vi "test.vi"() -> ()   [LabVIEW 2017]
uses:
  <vilib>/Analysis/NI_AALBase.lvlib
panel:
  out "Цифровой сигнал с паузами 3":dbl[][](graph)
  in  "Кол-во выборок":i32=400
  in  "Циклов в секунду\n(Модуляция)":i32(slide) scale=0.0..10.0
  out "Цифровой сигнал с паузами 2":dbl[][](graph)
  out "Waveform Graph":dbl[](graph)
  in  "Количество бит":i32=8
  out "Биты на выходе 1":dbl[](array[numeric])
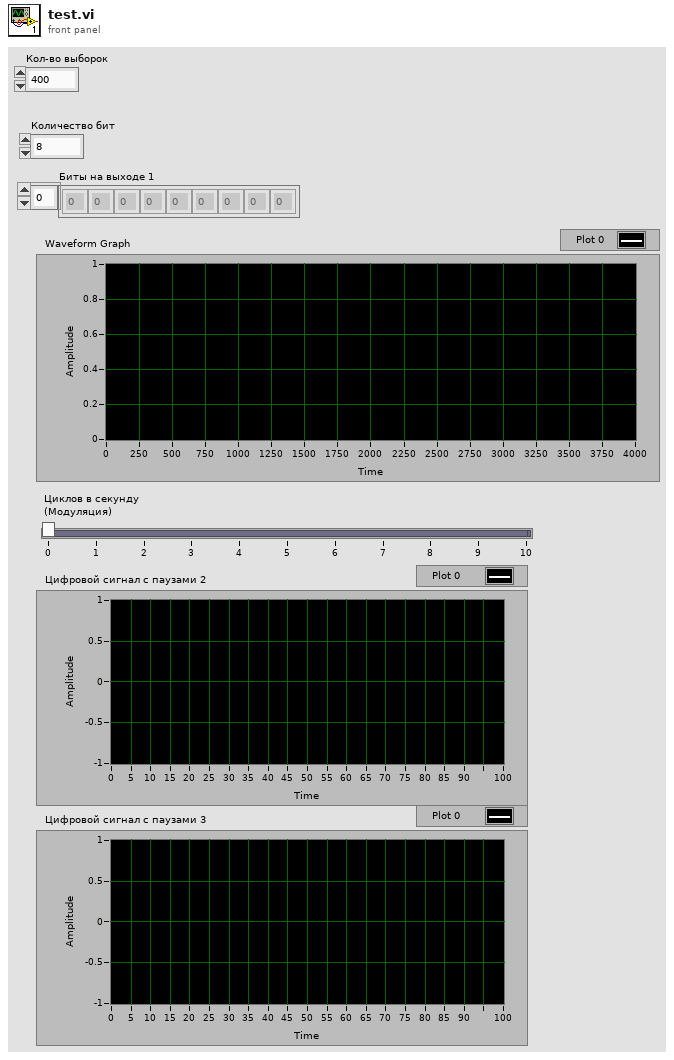
[diagram p1: front panel]
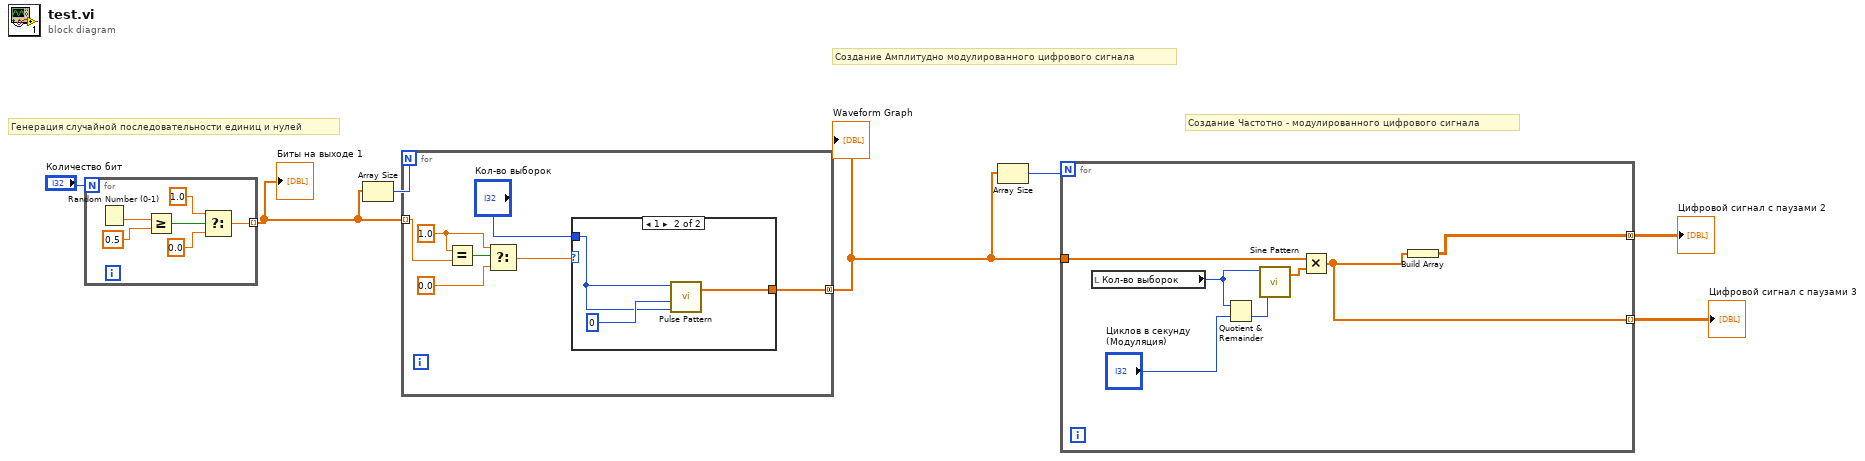
[diagram p0: block diagram]
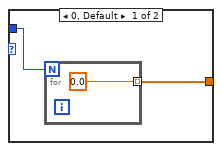
[diagram p2: hidden frame]
diagram:
  # "Создание Частотно - модулированного цифрового сигнала"
  # "Создание Амплитудно модулированного цифрового сигнала"
  # "Генерация случайной последовательности единиц и нулей"
  n1 = for {
    N: "Количество бит" -> [_]
    tunnel: [w8] -> w6 mode=indexing
    n2 = Random Number (0-1)() -> (number: 0 to 1=w13:dbl)
    n3 = Greater Or Equal?(x=w13, y=0.5) -> (x >= y?=w11:bool)
    n4 = Select(t=1.0, s=w11, f=0.0) -> (s? t:f=w8:dbl)
  }
  "Биты на выходе 1" <- w6
  n5 = Array Size(array=w6) -> (size(s)=w5:i32)
  n6 = for {
    N: w5 -> [_]
    tunnel: w6 -> [w17] mode=indexing
    tunnel: [w15] -> w3 mode=concatenating
    w19 = 1.0
    n7 = Equal?(x=w19, y=w17) -> (x = y?=w20:bool)
    n8 = Select(t=w19, s=w20, f=0.0) -> (s? t:f=w16:dbl)
    n9 = case shown="1" w16 {
      tunnel: [w21 w25] -> w15
      tunnel: "Кол-во выборок" -> [w22 w24]
      frame 0, Default {
        n10 = for {
          N: w22 -> [_]
          tunnel: [0.0] -> w21 mode=indexing
        }
      }
      frame 1 {
        n11 = call <vilib>:"Pulse Pattern.vi"("width"=w24, "delay"=0, "samples"=w24) -> ("Pulse Pattern"=w25:dbl[])  [unwired: 1 in, 1 out]
      }
    }
  }
  "Waveform Graph" <- w3
  n12 = Array Size(array=w3) -> (size(s)=w4:i32)
  n13 = for {
    N: w4 -> [_]
    tunnel: w3 -> [w29]
    tunnel: [w28] -> w2 mode=indexing
    tunnel: [w27] -> w1 mode=concatenating
    n14 = local read "Кол-во выборок"() -> (w31:i32)
    n15 = Quotient & Remainder(x=w31, y="Циклов в секунду\n(Модуляция)") -> (floor(x/y)=w32:i32)  [unwired: 1 out]
    n16 = call <vilib>:"Sine Pattern.vi"("cycles"=w32, "samples"=w31) -> ("Sinusoidal Pattern"=w33:dbl[])  [unwired: 2 in, 1 out]
    n17 = Multiply(x=w29, y=w33) -> (x*y=w28:dbl[])
    n18 = Build Array(w28) -> (w27:dbl[][])
  }
  "Цифровой сигнал с паузами 3" <- w2
  "Цифровой сигнал с паузами 2" <- w1
